vi "Configure.vi"(8 "error in (no error)":errorcluster, 11 "wavefront sensor in":refnum<class "wavefront sensor.lvclass">) -> (0 "error out":errorcluster, 2 "cancelled?":bool, 3 "wavefront sensor out":refnum<class "wavefront sensor.lvclass">)   [LabVIEW 2012, in "wavefront sensor.lvclass"]
doc: "The configure method configures the details for the RabbitMQ connection, the observers and the mapping script.\n\nIn the derived class, make a call to the parent for setting these parameters."
uses:
  wavefront sensor.lvclass
  <vilib>/Distrio/Murmex/Murmex/Murmex.lvclass
panel:
  # "RabbitMQ parameters"
  # "Window position"
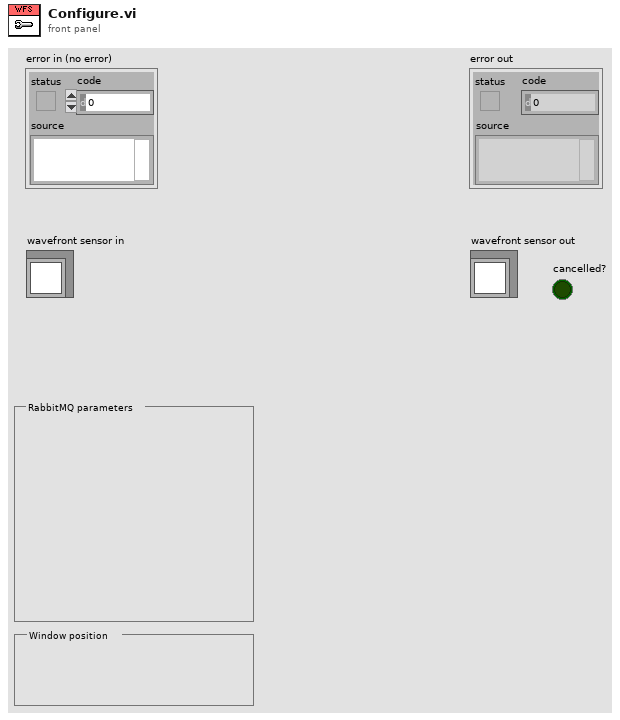
[diagram p1: front panel]
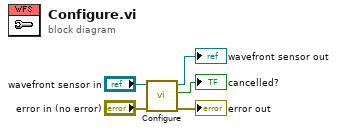
[diagram p0: block diagram]
diagram:
  n1 = call-parent "Configure.vi"("error in (no error)"="error in (no error)", "Murmex in"="wavefront sensor in") -> ("error out"=→"error out":errorcluster, "cancelled?"=→"cancelled?":bool, "Murmex out"=→"wavefront sensor out":refnum<class "wavefront sensor.lvclass">)  [unwired: 7 in]
